vi "Get Path Regex.vi"(8 "error in (no error)":errorcluster, 11 "CSRF in":refnum<class "CSRF.lvclass">) -> (0 "error out":errorcluster, 2 "Path Regex":string, 3 "CSRF out":refnum<class "CSRF.lvclass">)   [LabVIEW 2020, in "Summer of LabVIEW.lvlib" / "CSRF.lvclass"]
uses:
  CSRF.lvclass
  CSRF.lvclass/CSRF.ctl
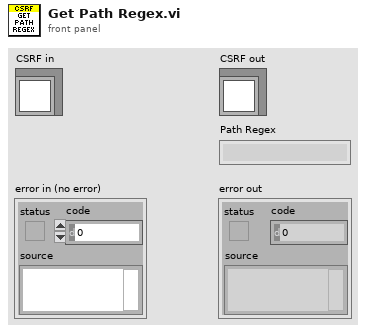
[diagram p1: front panel]
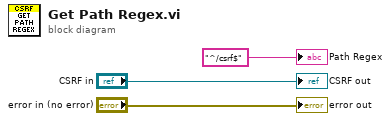
[diagram p0: block diagram]
diagram:
  "error out" <- "error in (no error)"
  "CSRF out" <- "CSRF in"
  "Path Regex" <- "^/csrf$" ("Path Regex")
